vi "波形图的游标与注释.vi"() -> ()   [LabVIEW 2014]
panel:
  out "data":dynamicdata(graph) caption="数据"
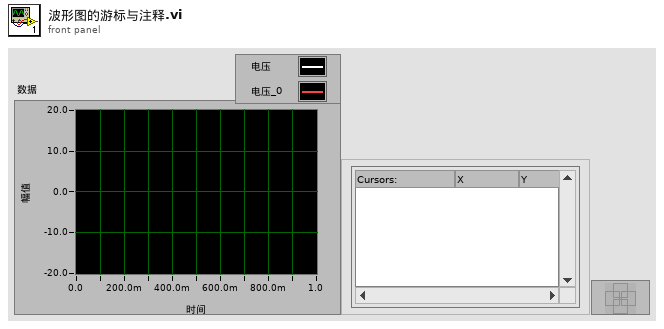
[diagram p1: front panel]
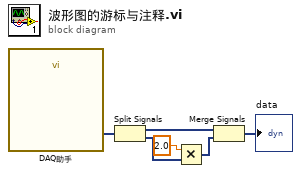
[diagram p0: block diagram]
diagram:
  n1 = call "DAQ助手"() -> ("data"=w6:dynamicdata)  [unwired: 17 in, 2 out]
  n2 = Split Signals(w6) -> (w3:dynamicdata, w5:dynamicdata)  [unwired: 2 in]
  n3 = Multiply(x=2.0, y=w5) -> (x*y=w4:dynamicdata)
  n4 = Merge Signals(w3, w4) -> (→"data":dynamicdata)
